vi "GlobalBin2x.vi"() -> ()   [LabVIEW 2010]
panel:
  out "Bin by 2":bool
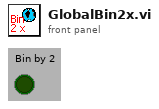
[diagram p1: front panel]
diagram:
